vi "Write Roles.vi"(8 "error in (no error)":errorcluster, 10 "Roles":T1, 11 "TestPlay in":refnum<class "TestPlay.lvclass">) -> (0 "error out":errorcluster, 3 "TestPlay out":refnum<class "TestPlay.lvclass">)   [LabVIEW 2023, in "TestPlay.lvclass"]
uses:
  TestPlay.lvclass
  TestRole_class/TestRole.lvclass
  Role_class/Role.lvclass
  SupportAttackerRole/SupportAttackerRole.lvclass
  TestPlay.lvclass/TestPlay.ctl
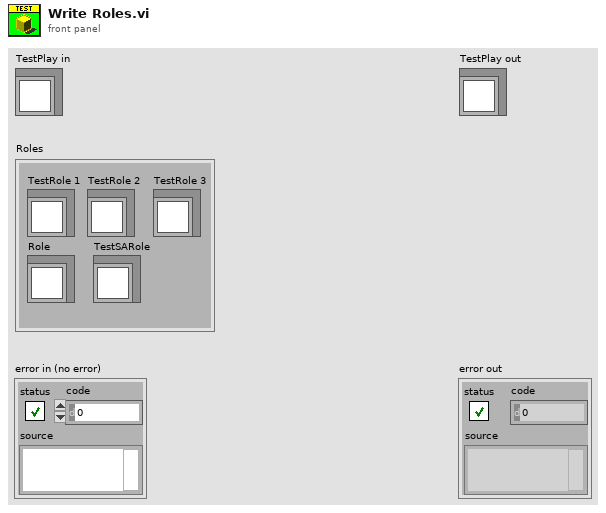
[diagram p1: front panel]
types:
  T1 = cluster{"TestRole 1":refnum<class "TestRole.lvclass">, "Role":refnum<class "Role.lvclass">, "TestRole 2":refnum<class "TestRole.lvclass">, "TestRole 3":refnum<class "TestRole.lvclass">, "TestSARole":refnum<class "SupportAttackerRole.lvclass">}
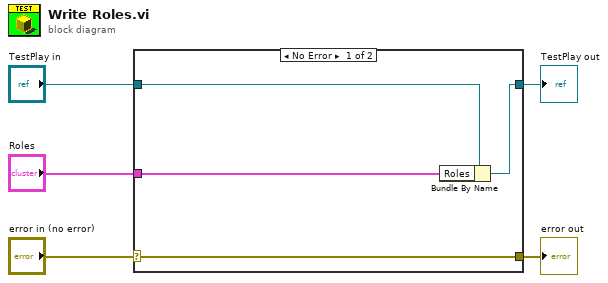
[diagram p0: block diagram]
diagram:
  n1 = case shown="No Error" "error in (no error)" {
    selector: "error in (no error)" -> [w9 w10]
    tunnel: [w9 w10] -> w4
    tunnel: [w7 w11] -> w2
    tunnel: "TestPlay in" -> [w8 w11]
    tunnel: "Roles" -> [w6 _]
    frame No Error {
      n2 = Bundle By Name(cluster=w8, "Roles"=w6) -> (w7:refnum<class "TestPlay.lvclass">)
    }
    frame Error {
    }
  }
  "error out" <- w4
  "TestPlay out" <- w2
